vi "Resize AOI on list.vi"(2 "New y dimension":u16, 3 "New x dimension":u16, 4 "Coordinates of  AOI to resize":u16[](array[numeric])) -> ()   [LabVIEW 2011]
doc: "Resize the AOI in the AOI list which is closest to the x and y coordinates given. The AOI center is kept at the same place, but its dimensions are adjusted to those specified."
uses:
  AOI List Globals.vi
panel:
  out "AOI number of resized AOI":i32
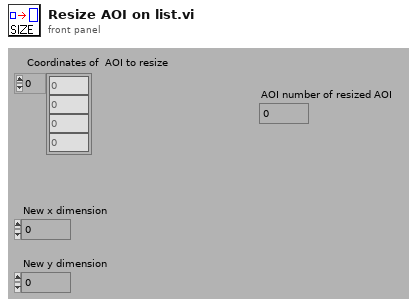
[diagram p1: front panel]
types:
  T1 = cluster{"AOI List[0]":u16, "AOI List[1]":u16, "AOI List[2]":u16, "AOI List[3]":u16}
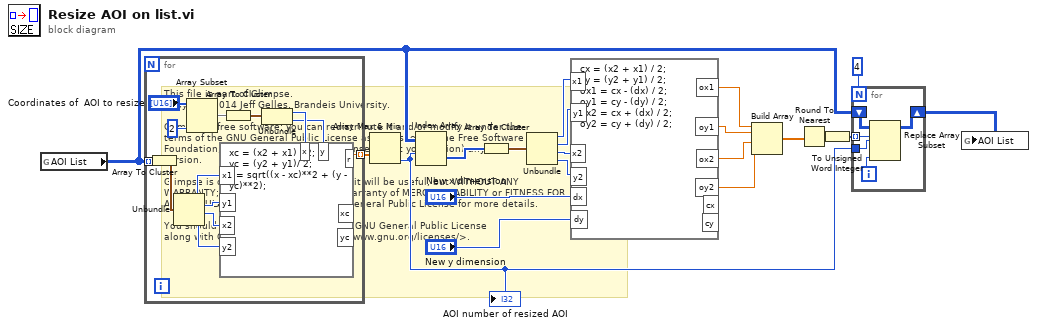
[diagram p0: block diagram]
diagram:
  # "This file is part of Glimpse. \nCopyright 2014 Jeff Gelles, Brandeis University.    \n\nGlimpse is free software: you can redistribute it and/or modify it under the \nterms of the GNU General Public License as published by the Free Software \nFoundation, either version 3 of the License, or (at your option) any later \nversion.\n\nGlimpse is distributed in the hope that it will be useful, but WITHOUT ANY \nWARRANTY; without even the implied warranty of MERCHANTABILITY or FITNESS FOR \nA PARTICULAR PURPOSE.  See the GNU General Public License for more details.\n\nYou should have received a copy of the GNU General Public License\nalong with Glimpse.  If not, see <http://www.gnu.org/licenses/>."
  n1 = global read "AOI List Globals.vi" "AOI List"() -> (w3:u16[][])
  n2 = for {
    tunnel: w3 -> [w27] mode=indexing
    tunnel: [w21] -> w2 mode=indexing
    n3 = Array To Cluster(array=w27) -> (cluster=w26:T1)
    n4 = Unbundle(w26) -> ("AOI List[0]"=w25:u16, "AOI List[1]"=w23:u16, "AOI List[2]"=w22:u16, "AOI List[3]"=w24:u16)
    n5 = Array Subset(array="Coordinates of  AOI to resize", length=2) -> (w31:u16[])  [unwired: 1 in]
    n6 = Array To Cluster(array=w31) -> (cluster=w30:cluster{"[0]":u16, "[1]":u16})
    n7 = Unbundle(w30) -> ("[0]"=w29:u16, "[1]"=w28:u16)
    n8 = formula code="xc = (x2 + x1) / 2;\nyc = (y2 + y1)/ 2;\nr = sqrt((x - xc)**2 + (y - yc)**2);"("x"=w29, "y"=w28, "x1"=w25, "y1"=w23, "x2"=w22, "y2"=w24) -> ("r"=w21:dbl)  [unwired: 2 out]
  }
  n9 = Array Max & Min(array=w2) -> (min index (indices)=w6:i32)  [unwired: 3 out]
  "AOI number of resized AOI" <- w6
  n10 = Index Array(array=w3, index (row)=w6) -> (element=w19:u16[])  [unwired: 1 in]
  n11 = Array To Cluster(array=w19) -> (cluster=w20:T1)
  n12 = Unbundle(w20) -> ("AOI List[0]"=w15:u16, "AOI List[1]"=w16:u16, "AOI List[2]"=w17:u16, "AOI List[3]"=w18:u16)
  n13 = formula code="cx = (x2 + x1) / 2;\ncy = (y2 + y1) / 2;\nox1 = cx - (dx) / 2;\noy1 = cy - (dy) / 2;\nox2 = cx + (dx) / 2;\noy2 = cy + (dy) / 2;"("x2"=w17, "x1"=w15, "y1"=w16, "y2"=w18, "dx"="New x dimension", "dy"="New y dimension") -> ("ox1"=w9:dbl, "oy1"=w10:dbl, "ox2"=w11:dbl, "oy2"=w12:dbl)  [unwired: 2 out]
  n14 = Build Array(w9, w10, w11, w12) -> (w8:dbl[])
  n15 = Round To Nearest(number=w8) -> (nearest integer value=w7:dbl[])
  n16 = To Unsigned Word Integer(number=w7) -> (unsigned 16bit integer=w1:u16[])
  n17 = for {
    N: 4 -> [_]
    tunnel: w1 -> [w38] mode=indexing
    tunnel: w6 -> [w37]
    shift-right: [w34] -> w4
    shift-left: w3 -> [w35]
    i -> [w36]
    n18 = Replace Array Subset(array=w35, new element=w38, index (row)=w37, index (col)=w36) -> (w34:u16[][])
  }
  n19 = global write "AOI List Globals.vi" "AOI List"(w4) -> ()
